vi "Get IDs or Error.vi"(0 "IHandlePublished in":refnum<class "IHandlePublished.lvclass">, 11 "error in (no error)":errorcluster) -> (4 "IHandlePublished out":refnum<class "IHandlePublished.lvclass">, 6 "Publish request ID":u64, 8 "Publication ID":u64, 10 "ErrorOrSuccess":refnum<class "ErrorOrSuccess.lvclass">, 15 "error out":errorcluster)   [LabVIEW 2020, in "wamplv.lvlib" / "IHandlePublished.lvclass"]
uses:
  IHandlePublished.lvclass
  Message loop classes/ErrorOrSuccess/ErrorOrSuccess.lvclass
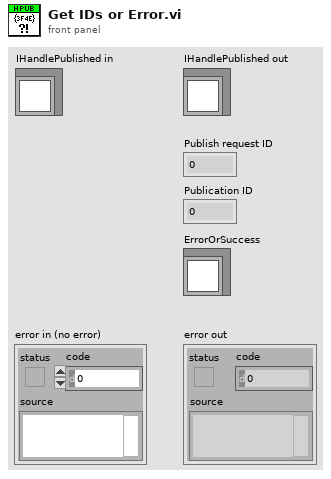
[diagram p1: front panel]
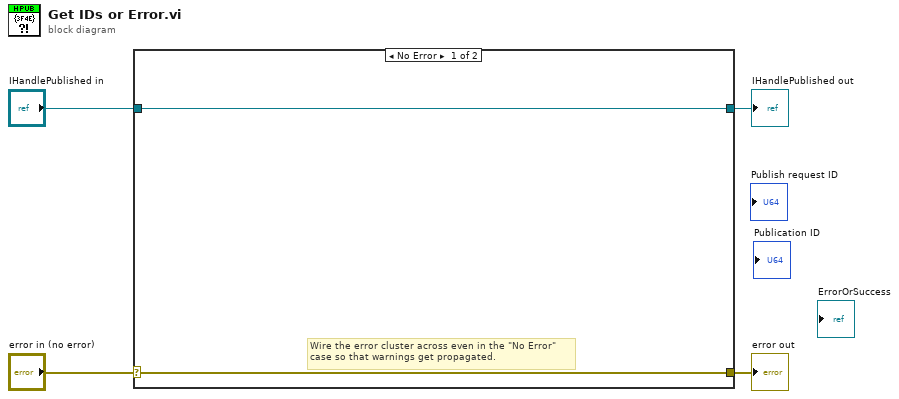
[diagram p0: block diagram]
diagram:
  n1 = case shown="No Error" "error in (no error)" {
    selector: "error in (no error)" -> [w5 w8]
    tunnel: [w5 w8] -> w3
    tunnel: [w6 w7] -> w1
    tunnel: "IHandlePublished in" -> [w6 w7]
    frame No Error {
      # "Wire the error cluster across even in the \"No Error\"\ncase so that warnings get propagated."
    }
    frame Error {
    }
  }
  "error out" <- w3
  "IHandlePublished out" <- w1
